vi "Main.vi"() -> ()   [LabVIEW 2015]
uses:
  <vilib>/Utility/error.llb/DialogType.ctl
panel:
  out "Conn status":bool caption="Connected"
  out "Spellman out, кВ":string
  in  "k":dbl=20.0 min=-10.0 max=100.0 step=0.001 format="%#.3f"
  in  "выкл.":bool
  in  "IP":string="172.16.21.207"
  in  "SetRemote":bool
  in  "Сброс ERR":bool
  in  "График":bool=TRUE
  in  "Current":u16 caption="мА" max=30 step=1
  in  "SetIB":bool
  in  "Voltage":dbl=0.01 caption="кВ" min=0.001 max=149.999 step=0.001 format="%06.3f"
  in  "SetUB":bool
  out "Режим":bool
  out "Статус":bool
  out "Блокировка":bool
  out "мА":string
  out "Output":bool
  in  "вкл.":bool
  out "conn src":refnum<k5>
  in  "stop":bool
  out "message":string=" INSTRUCTIONS:\r\rNormal Use:  When using subVIs that incorporate the error in/error out (or error I/O) structure, place this handler where you want to inform the user of an error, typically at the end of the I/O data path, as the last action of the program.  If the error in error? is ERROR, the handler creates a message describing the error and its source.  If the type of dialog = 1 (default), the message is displayed to the user, who can only acknowedge it.  If the type = 2, the user can acknowledge the message or abort execution; aborting a program with active I/O is not recommended.  If the type = 0, no message is displayed; this is used to process the error programmatically, and the error out cluster elements are wired to individual terminals for that reason.  \r\rOther Use:\n\r\nlocal testing.  To test the error code of a subVI or function that does not have the error I/O structure, you can wire its error code and a source string to the local error code and error source inputs.  If error in error? indicates no error and error code is not equal to 0, the local code and source are substituted for the error in values, and error? is set TRUE (ERROR)."
  out "кВ":string
  out "Uвых":dbl(graph)
  # "ИТ 150         SPELLMAN 10 кВ 30 мА"
  # "Settings"
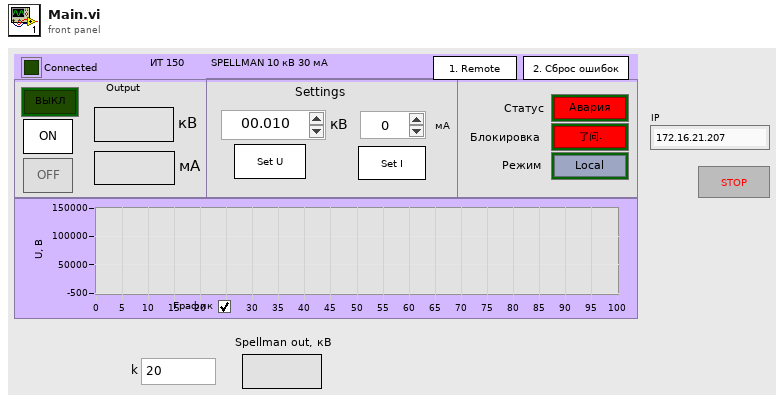
[diagram p1: front panel]
types:
  T1 = enum16{"open", "replace", "create", "open or create", "replace or create", "replace or create with confirmation"}
  T2 = typedef "DialogType.ctl" = u16
  T3 = enum8{"Enabled", "Disabled", "Disabled and Grayed Out"}
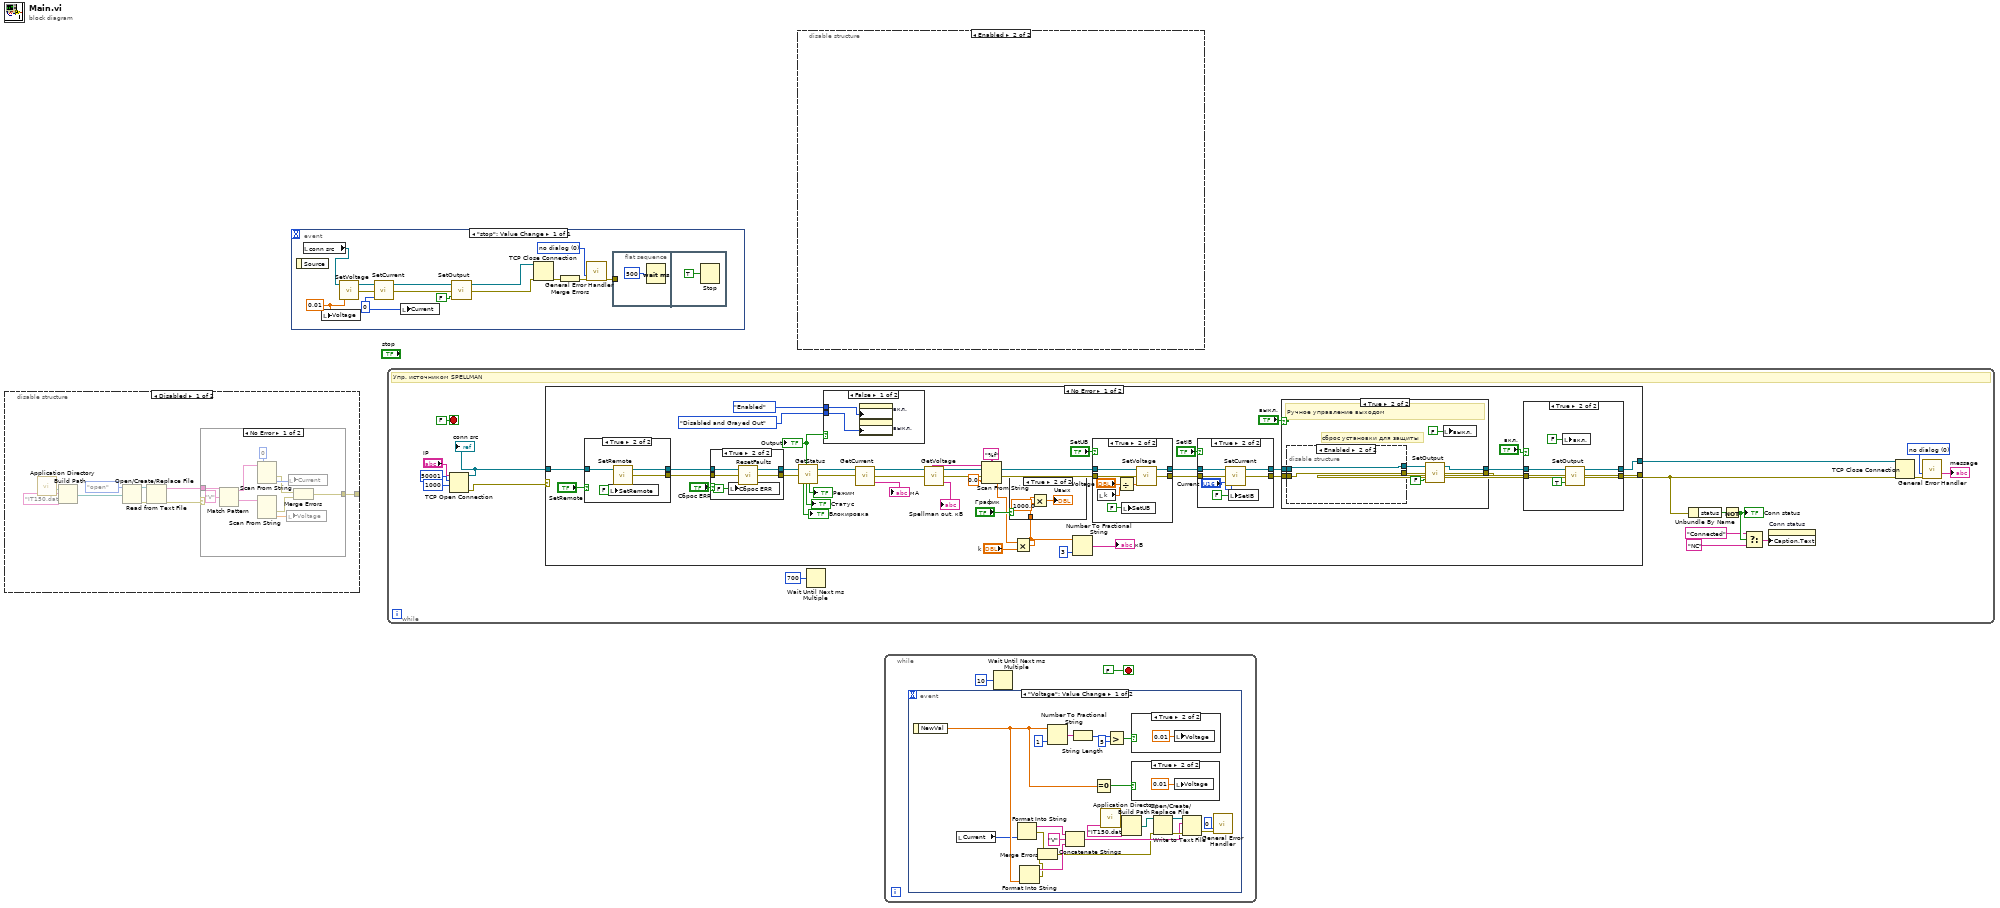
[diagram p0: block diagram]
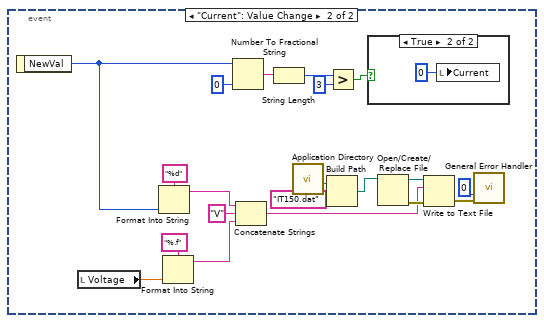
[diagram p6: hidden frame]
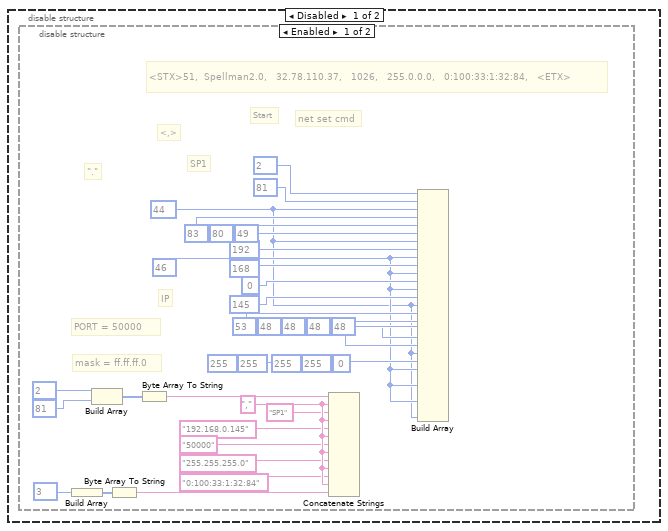
[diagram p8: hidden frame]
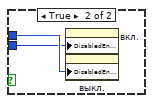
[diagram p10: hidden frame]
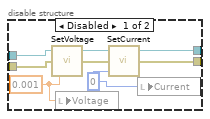
[diagram p18: hidden frame]
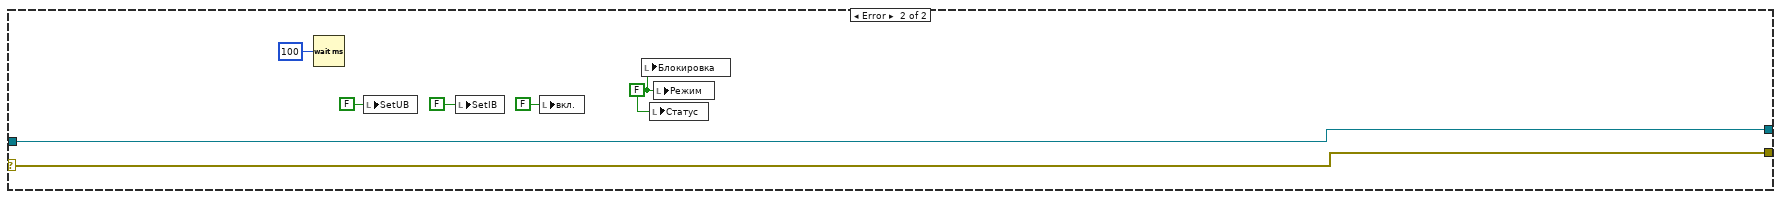
[diagram p19: hidden frame]
diagram:
  n1 = disable-structure shown="Disabled" {
    disable-tunnel: [w2 _] -> _
    frame Disabled {
      n2 = call <vilib>:"Application Directory.vi"() -> ("Application Directory"=w3:path)
      n3 = Build Path(base path=w3, name or relative path="IT150.dat") -> (appended path=w6:path)
      n4 = Open/Create/Replace File(file path (use dialog)=w6, operation (0:open)=T1."open") -> (refnum out=w8:refnum<file>, error out=w7:errorcluster)  [unwired: 4 in, 1 out]
      n5 = Read from Text File(file (use dialog)=w8, error in=w7) -> (text=w9:string, error out=w1:errorcluster)  [unwired: 2 in, 2 out]
      n6 = case shown="No Error" w1 {
        selector: w1 -> [_ w20]
        tunnel: w9 -> [w16 _]
        tunnel: [w10 w20] -> w2
        frame No Error {
          n7 = Match Pattern(string=w16, regular expression="V" ("string")) -> (before substring=w17:string, after substring=w19:string)  [unwired: 1 in, 2 out]
          n8 = Scan From String(input string=w17, default 1=u16 0 ("default value 1")) -> (error out=w12:errorcluster, output 1=w13:u16)  [unwired: 3 in, 2 out]
          n9 = Scan From String(input string=w19) -> (error out=w11:errorcluster, output 1=w14:dbl)  [unwired: 4 in, 2 out]
          n10 = local write "Voltage"(w14) -> ()
          n11 = local write "Current"(w13) -> ()
          n12 = Merge Errors(w12, w11) -> (w10:errorcluster)
        }
        frame Error {
        }
      }
    }
    frame Enabled {
    }
  }
  n13 = event shown="[0] \"stop\": Value Change" {
    selector: _ -> [_]
    dyn-events: _ -> [_]
    timeout: _ -> [_]
    event "stop": Value Change {
      w21 = u16 0 ("Current")
      w22 = 0.01 ("Voltage")
      w32 = T2 0 items=["no dialog", "OK message", "continue or stop message", "OK message + warnings", "continue/stop + warnings"] ("type of dialog (OK msg:1)")
      n14 = event-data() -> ()  [unwired: 1 in, 1 out]
      n15 = local read "conn src"() -> (w25:refnum<k5>)
      n16 = local write "Voltage"(w22) -> ()
      n17 = call "SetVoltage.vi"("Voltage"=w22, "connection ID"=w25) -> ("error out"=w26:errorcluster, "connection ID out"=w27:refnum<k5>)  [unwired: 1 in, 1 out]
      n18 = call "SetCurrent.vi"("Current"=w21, "error in"=w26, "connection ID in"=w27) -> ("error out"=w28:errorcluster, "connection ID out"=w29:refnum<k5>)  [unwired: 1 out]
      n19 = local write "Current"(w21) -> ()
      n20 = call "SetOutput.vi"("State"=FALSE, "error in"=w28, "connection ID"=w29) -> ("error out"=w23:errorcluster, "connection ID out"=w24:refnum<k5>)  [unwired: 1 in]
      n21 = TCP Close Connection(connection ID=w24, error in (no error)=w23) -> (error out=w34:errorcluster)  [unwired: 1 in, 1 out]
      n22 = Merge Errors(w34) -> (w33:errorcluster)
      n23 = call <vilib>:"General Error Handler.vi"("type of dialog (OK msg:1)"=w32, "error in (no error)"=w33) -> ("error out"=w31:errorcluster)  [unwired: 9 in, 4 out]
      n24 = flat-sequence {
        tunnel: w31 -> [_]
        frame #0 {
          n25 = Wait (ms)(milliseconds to wait=u32 500) -> ()  [unwired: 1 out]
        }
        frame #1 {
          n26 = Stop(stop? (T)=TRUE) -> ()
        }
      }
    }
  }
  n27 = while {
    stop <- FALSE stop-if-true
    w52 = T2 0 items=["no dialog", "OK message", "continue or stop message", "OK message + warnings", "continue/stop + warnings"] ("type of dialog (OK msg:1)")
    # "Упр. источником SPELLMAN"
    n28 = TCP Open Connection(address="IP", remote port or service name=u16 50001 ("Port"), timeout ms (60000)=1000) -> (connection ID=w46:refnum<k5>, error out=w45:errorcluster)  [unwired: 2 in]
    "conn src" <- w46
    n29 = case shown="No Error" w45 {
      selector: w45 -> [_ w165]
      tunnel: w46 -> [w71 w166]
      tunnel: [w65 w166] -> w43
      tunnel: [w64 w165] -> w42
      frame No Error {
        n30 = case shown="True" "SetRemote" {
          tunnel: [w108 w112] -> w72
          tunnel: w71 -> [w108 w111]
          tunnel: [_ w110] -> w70
          frame False {
          }
          frame True {
            n31 = local write "SetRemote"(FALSE ("SetRemote")) -> ()
            n32 = call "SetRemote.vi"("connection ID"=w111) -> ("error out"=w110:errorcluster, "connection ID out"=w112:refnum<k5>)  [unwired: 2 in, 1 out]
          }
        }
        n33 = case shown="True" "Сброс ERR" {
          tunnel: w72 -> [w114 w119]
          tunnel: [w114 w118] -> w73
          tunnel: [w113 w117] -> w74
          tunnel: w70 -> [w113 w115]
          frame False {
          }
          frame True {
            n34 = local write "Сброс ERR"(FALSE ("Сброс ERR")) -> ()
            n35 = call "ResetFaults.vi"("error in"=w115, "connection ID"=w119) -> ("error out"=w117:errorcluster, "connection ID out"=w118:refnum<k5>)  [unwired: 1 in, 1 out]
          }
        }
        n36 = call "GetStatus.vi"("connection ID in"=w73, "error in"=w74) -> ("InterlLoc State"=→"Блокировка":bool, "OutState"=w62:bool, "Fault"=→"Статус":bool, "Rem|Loc"=→"Режим":bool, "connection ID out"=w80:refnum<k5>, "error out"=w79:errorcluster)  [unwired: 12 in]
        "Output" <- w62
        n37 = case shown="False" w62 {
          tunnel: T3."Enabled" ("Disabled") -> [w97 w99]
          tunnel: T3."Disabled and Grayed Out" ("Disabled") -> [w96 w98]
          frame False {
            n38 = property on="вкл." class="Bool (strict)"("DisabledEnum"=w97) -> ()  [unwired: 2 in, 2 out]
            n39 = property on="выкл." class="Bool (strict)"("DisabledEnum"=w96) -> ()  [unwired: 2 in, 2 out]
          }
          frame True {
            n40 = property on="вкл." class="Bool (strict)"("DisabledEnum"=w98) -> ()  [unwired: 2 in, 2 out]
            n41 = property on="выкл." class="Bool (strict)"("DisabledEnum"=w99) -> ()  [unwired: 2 in, 2 out]
          }
        }
        n42 = call "GetCurrent.vi"("error in"=w79, "connection ID"=w80) -> ("Current"=→"мА":string, "error out"=w95:errorcluster, "connection ID out"=w94:refnum<k5>)  [unwired: 1 out]
        n43 = call "GetVoltage.vi"("error in"=w95, "connection ID"=w94) -> ("Voltage"=w55:string, "error out"=w88:errorcluster, "connection ID out"=w93:refnum<k5>)  [unwired: 1 out]
        "Spellman out, кВ" <- w55
        n44 = Scan From String(format string="%f", input string=w55, error in=w88, default 1=0.0 ("default (0 I32)")) -> (error out=w87:errorcluster, output 1=w58:dbl)  [unwired: 1 in, 2 out]
        n45 = Multiply(x=w58, y="k") -> (x*y=w56:dbl)
        n46 = case shown="True" "График" {
          tunnel: w56 -> [_ w120]
          frame False {
          }
          frame True {
            n47 = Multiply(x=w120, y=1000.0) -> (x*y=→"Uвых":dbl)
          }
        }
        n48 = Number To Fractional String(number=w56, precision (6)=i16 3) -> (F-format string=→"кВ":string)  [unwired: 2 in]
        n49 = case shown="True" "SetUB" {
          tunnel: w87 -> [w132 w140]
          tunnel: [w132 w139] -> w84
          tunnel: w93 -> [w131 w138]
          tunnel: [w131 w136] -> w85
          frame False {
          }
          frame True {
            n50 = local read "k"() -> (w134:dbl)
            n51 = Divide(x="Voltage", y=w134) -> (x/y=w133:dbl)
            n52 = local write "SetUB"(FALSE ("SetUB")) -> ()
            n53 = call "SetVoltage.vi"("Voltage"=w133, "error in"=w140, "connection ID"=w138) -> ("error out"=w139:errorcluster, "connection ID out"=w136:refnum<k5>)  [unwired: 1 out]
          }
        }
        n54 = case shown="True" "SetIB" {
          tunnel: w85 -> [w124 w129]
          tunnel: w84 -> [w123 w128]
          tunnel: [w123 w127] -> w83
          tunnel: [w124 w126] -> w82
          frame False {
          }
          frame True {
            n55 = call "SetCurrent.vi"("Current"="Current", "error in"=w128, "connection ID in"=w129) -> ("error out"=w127:errorcluster, "connection ID out"=w126:refnum<k5>)  [unwired: 1 out]
            n56 = local write "SetIB"(FALSE ("SetUB")) -> ()
          }
        }
        n57 = case shown="True" "выкл." {
          tunnel: [w142 w144] -> w68
          tunnel: [w141 w145] -> w63
          tunnel: w83 -> [w141 w147]
          tunnel: w82 -> [w142 w146]
          frame False {
          }
          frame True {
            # "сброс установки для защиты"
            # "Ручное управление выходом"
            n58 = disable-structure shown="Enabled" {
              disable-tunnel: [w158 w160] -> w149
              disable-tunnel: [w157 w159] -> w148
              disable-tunnel: w147 -> [w154 w159]
              disable-tunnel: w146 -> [w153 w160]
              frame Disabled {
                w151 = u16 0 ("Current")
                w152 = 0.001 ("Voltage")
                n59 = call "SetVoltage.vi"("Voltage"=w152, "error in"=w154, "connection ID"=w153) -> ("error out"=w155:errorcluster, "connection ID out"=w156:refnum<k5>)  [unwired: 1 out]
                n60 = local write "Voltage"(w152) -> ()
                n61 = call "SetCurrent.vi"("Current"=w151, "error in"=w155, "connection ID in"=w156) -> ("error out"=w157:errorcluster, "connection ID out"=w158:refnum<k5>)  [unwired: 1 out]
                n62 = local write "Current"(w151) -> ()
              }
              frame Enabled {
              }
            }
            n63 = call "SetOutput.vi"("State"=FALSE, "error in"=w148, "connection ID"=w149) -> ("error out"=w145:errorcluster, "connection ID out"=w144:refnum<k5>)  [unwired: 1 in]
            n64 = local write "выкл."(FALSE ("выкл.")) -> ()
          }
        }
        n65 = case shown="True" "вкл." {
          tunnel: w68 -> [w101 w107]
          tunnel: [w101 w106] -> w65
          tunnel: [w100 w105] -> w64
          tunnel: w63 -> [w100 w104]
          frame False {
          }
          frame True {
            n66 = local write "вкл."(FALSE ("вкл.")) -> ()
            n67 = call "SetOutput.vi"("State"=TRUE, "error in"=w104, "connection ID"=w107) -> ("error out"=w105:errorcluster, "connection ID out"=w106:refnum<k5>)  [unwired: 1 in]
          }
        }
      }
      frame Error {
        w161 = FALSE ("Режим")
        n68 = Wait (ms)(milliseconds to wait=u32 100) -> ()  [unwired: 1 out]
        n69 = local write "SetUB"(FALSE ("SetUB")) -> ()
        n70 = local write "SetIB"(FALSE ("SetUB")) -> ()
        n71 = local write "вкл."(FALSE ("вкл.")) -> ()
        n72 = local write "Блокировка"(w161) -> ()
        n73 = local write "Статус"(w161) -> ()
        n74 = local write "Режим"(w161) -> ()
      }
    }
    n75 = Wait Until Next ms Multiple(millisecond multiple=u32 700 ("milliseconds to wait")) -> ()  [unwired: 1 out]
    n76 = Unbundle By Name(w42) -> ("status"=w41:bool)
    n77 = Not(x=w41) -> (.not. x?=w40:bool)
    "Conn status" <- w40
    n78 = Select(t="Connected", s=w40, f="NC") -> (s? t:f=w39:string)
    n79 = property on="Conn status" class="Bool (strict)"("Caption.Text"=w39) -> ()  [unwired: 2 in, 2 out]
    n80 = TCP Close Connection(connection ID=w43, error in (no error)=w42) -> (error out=w53:errorcluster)  [unwired: 2 out]
    n81 = call <vilib>:"General Error Handler.vi"("type of dialog (OK msg:1)"=w52, "error in (no error)"=w53) -> ("message"=→"message":string)  [unwired: 9 in, 4 out]
  }
  n82 = disable-structure shown="Enabled" {
    frame Disabled {
      n83 = disable-structure shown="Enabled" {
        frame Enabled {
          w177 = "," ("string")
          (unwired) u8 0 ("y")
          (unwired) u8 255 ("y")
          (unwired) u8 255 ("y")
          (unwired) u8 255 ("y")
          w182 = u8 46 ("y")
          w181 = u8 44 ("y")
          # "mask = ff.ff.ff.0"
          # "PORT = 50000"
          # "IP"
          # "\".\""
          # "net set cmd"
          # "Start"
          # "<,>"
          # "SP1"
          # "<STX>51,  Spellman2.0,   32.78.110.37,   1026,   255.0.0.0,   0:100:33:1:32:84,   <ETX>"
          n84 = Build Array(u8 3 ("y")) -> (w179:u8[])
          n85 = Build Array(u8 2 ("y"), u8 81 ("y")) -> (w168:u8[])
          n86 = Byte Array To String(unsigned byte array=w179) -> (string=w180:string)
          n87 = Byte Array To String(unsigned byte array=w168) -> (string=w171:string)
          n88 = Concatenate Strings(w171, w177, "SP1" ("string"), w177, "192.168.0.145", w177, "50000", w177, "255.255.255.0", w177, "0:100:33:1:32:84", w177, w180) -> ()  [unwired: 1 out]
          n89 = Build Array(u8 2 ("y"), u8 81 ("y"), w181, u8 83 ("y"), u8 80 ("y"), u8 49 ("y"), w181, u8 192 ("y"), w182, u8 168 ("y"), w182, u8 0 ("y"), w182, u8 145 ("y"), w181, u8 53 ("y"), u8 48 ("y"), u8 48 ("y"), u8 48 ("y"), u8 48 ("y"), w181, u8 255 ("y"), w182, w182, w182, w181) -> ()  [unwired: 3 in, 1 out]
        }
        frame Disabled {
        }
      }
    }
    frame Enabled {
    }
  }
  n90 = while {
    stop <- FALSE stop-if-true
    n91 = event shown="[0] \"Voltage\": Value Change" {
      selector: _ -> [_ _]
      dyn-events: _ -> [_ _]
      timeout: _ -> [_ _]
      event "Voltage": Value Change {
        n92 = event-data() -> ("NewVal"=w204:dbl)  [unwired: 1 in]
        n93 = local read "Current"() -> (w203:u16)
        n94 = Format Into String(w203) -> (resulting string=w214:string, error out=w202:errorcluster)  [unwired: 3 in]
        n95 = Format Into String(w204) -> (resulting string=w215:string, error out=w201:errorcluster)  [unwired: 3 in]
        n96 = Merge Errors(w202, w201) -> (w200:errorcluster)
        n97 = Number To Fractional String(number=w204, precision (6)=i16 1) -> (F-format string=w220:string)  [unwired: 2 in]
        n98 = Concatenate Strings(w214, "V" ("string"), w215) -> (w211:string)
        n99 = String Length(string=w220) -> (length=w219:i32)
        n100 = Equal To 0?(x=w204) -> (x = 0?=w216:bool)
        n101 = call <vilib>:"Application Directory.vi"() -> ("Application Directory"=w209:path)
        n102 = Greater?(x=w219, y=5) -> (0:w217:bool)
        n103 = Build Path(base path=w209, name or relative path="IT150.dat") -> (appended path=w208:path)
        n104 = case shown="True" w216 {
          frame False {
          }
          frame True {
            n105 = local write "Voltage"(0.01 ("Voltage")) -> ()
          }
        }
        n106 = case shown="True" w217 {
          frame False {
          }
          frame True {
            n107 = local write "Voltage"(0.01 ("Voltage")) -> ()
          }
        }
        n108 = Open/Create/Replace File(file path (use dialog)=w208, error in=w200) -> (refnum out=w213:refnum<file>, error out=w212:errorcluster)  [unwired: 4 in, 1 out]
        n109 = Write to Text File(file (use dialog)=w213, text=w211, error in=w212) -> (error out=w206:errorcluster)  [unwired: 1 in, 2 out]
        n110 = call <vilib>:"General Error Handler.vi"("type of dialog (OK msg:1)"=u32 0 ("milliseconds to wait"), "error in (no error)"=w206) -> ()  [unwired: 9 in, 5 out]
      }
      event "Current": Value Change {
        n111 = event-data() -> ("NewVal"=w225:u16)  [unwired: 1 in]
        n112 = local read "Voltage"() -> (w224:dbl)
        n113 = Format Into String(format string="%d", w225) -> (resulting string=w236:string)  [unwired: 2 in, 1 out]
        n114 = Format Into String(format string="%.f", w224) -> (resulting string=w238:string)  [unwired: 2 in, 1 out]
        n115 = Number To Fractional String(number=w225, precision (6)=i16 0) -> (F-format string=w242:string)  [unwired: 2 in]
        n116 = Concatenate Strings(w236, "V" ("string"), w238) -> (w232:string)
        n117 = String Length(string=w242) -> (length=w241:i32)
        n118 = call <vilib>:"Application Directory.vi"() -> ("Application Directory"=w230:path)
        n119 = Build Path(base path=w230, name or relative path="IT150.dat") -> (appended path=w229:path)
        n120 = Greater?(x=w241, y=3) -> (0:w239:bool)
        n121 = case shown="True" w239 {
          frame False {
          }
          frame True {
            n122 = local write "Current"(u16 0 ("Voltage")) -> ()
          }
        }
        n123 = Open/Create/Replace File(file path (use dialog)=w229) -> (refnum out=w234:refnum<file>, error out=w233:errorcluster)  [unwired: 5 in, 1 out]
        n124 = Write to Text File(file (use dialog)=w234, text=w232, error in=w233) -> (error out=w227:errorcluster)  [unwired: 1 in, 2 out]
        n125 = call <vilib>:"General Error Handler.vi"("type of dialog (OK msg:1)"=u32 0 ("milliseconds to wait"), "error in (no error)"=w227) -> ()  [unwired: 9 in, 5 out]
      }
    }
    n126 = Wait Until Next ms Multiple(millisecond multiple=u32 10 ("milliseconds to wait")) -> ()  [unwired: 1 out]
  }
